vi "LVClass_WavefrontCorrector set all WFC parameter values.vi"(0 "WavefrontCorrector in":refnum<class "WavefrontCorrector.lvclass">, 5 "AllWFCParametersValues":T1[](array[typedef]), 11 "error in (no error)":errorcluster) -> (4 "WavefrontCorrector out":refnum<class "WavefrontCorrector.lvclass">, 15 "error out":errorcluster)   [LabVIEW 2020, in "WavefrontCorrector.lvclass"]
uses:
  WavefrontCorrector.lvclass
  CameraParametersSetup.ctl
  CameraParameters_Type.ctl
  LVClass_WavefrontCorrector Read AllWavefrontCorrectorParametersProperties.vi
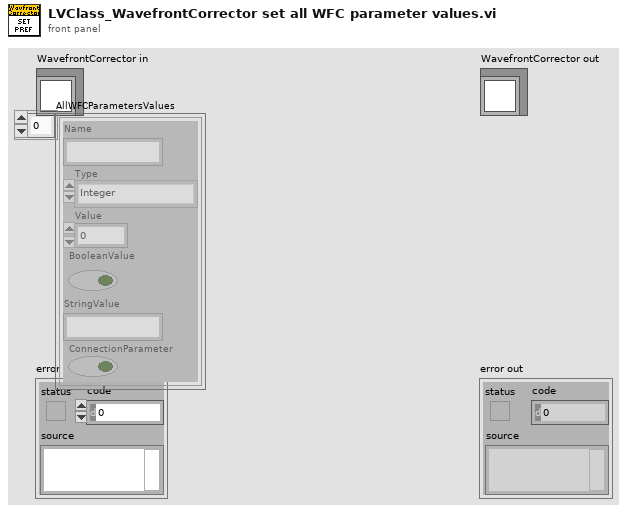
[diagram p1: front panel]
types:
  T1 = typedef "CameraParametersSetup.ctl" = cluster{"Name":string, "Type":T2, "Value":dbl, "BooleanValue":bool, "StringValue":string, "ConnectionParameter":bool}
  T2 = typedef "CameraParameters_Type.ctl" = enum16{"Integer", "Real", "String", "Boolean"}
  T3 = typedef "ParameterID.ctl" = cluster{"Name":string, "ConnectionParameter?":bool, "Type":T2, "Authorization":T4, "OnFlyAuthorization":T5, "StringValue":string, "Value":dbl, "Min":dbl, "Max":dbl, "BooleanValue":bool, "StringParameterList":string[]}
  T4 = typedef "CameraParameters_Authorization.ctl" = enum16{"Disable", "Gettable", "Settable - Gettable"}
  T5 = typedef "CameraParameters_OnFlyAuthorization.ctl" = enum16{"None", "Gettable", "Settable", "Settable - Gettable"}
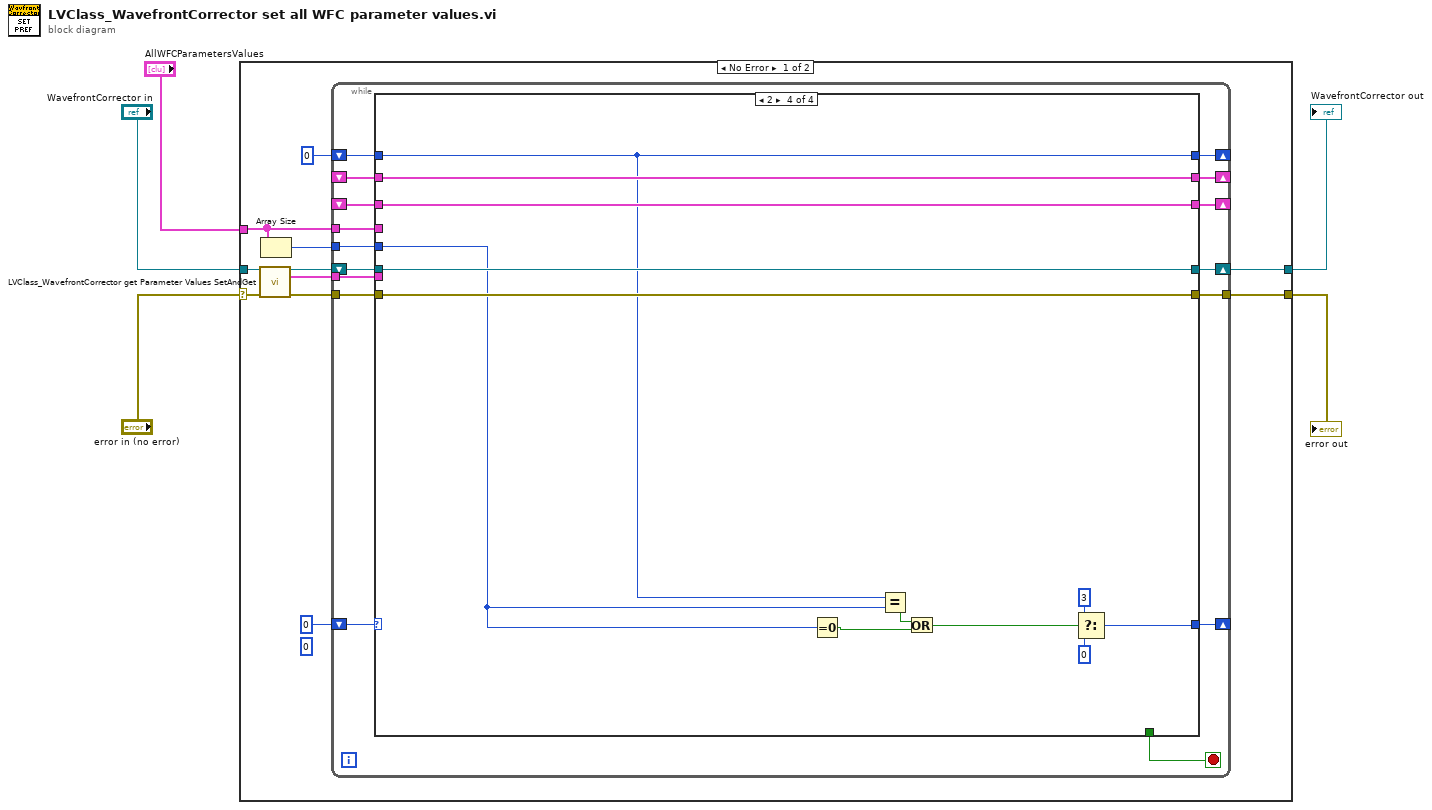
[diagram p0: block diagram]
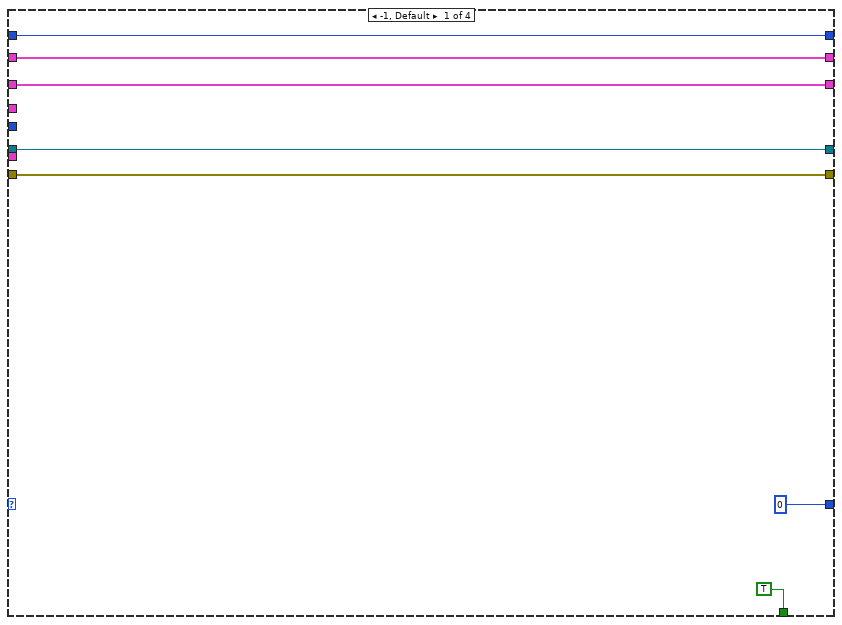
[diagram p2: hidden frame]
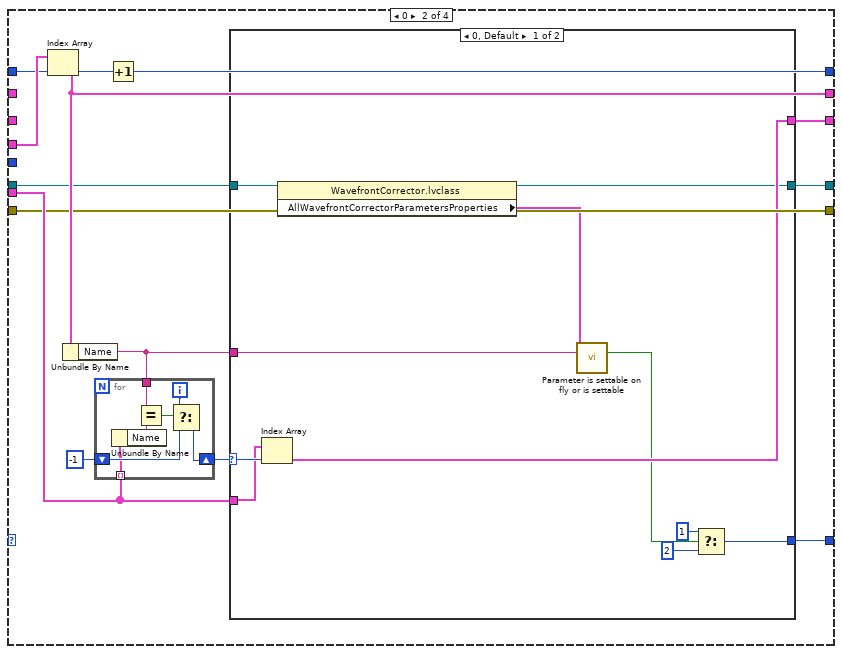
[diagram p3: hidden frame]
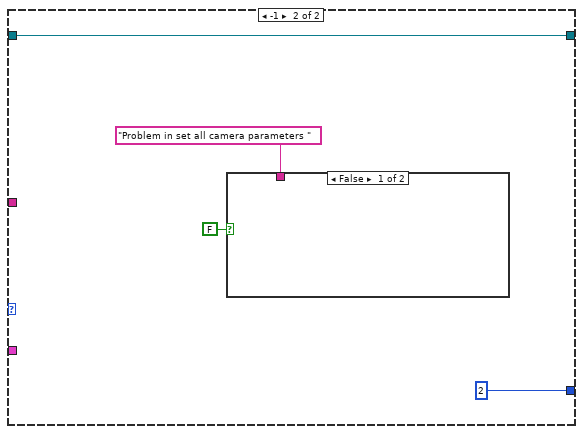
[diagram p4: hidden frame]
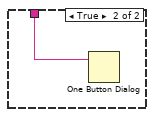
[diagram p5: hidden frame]
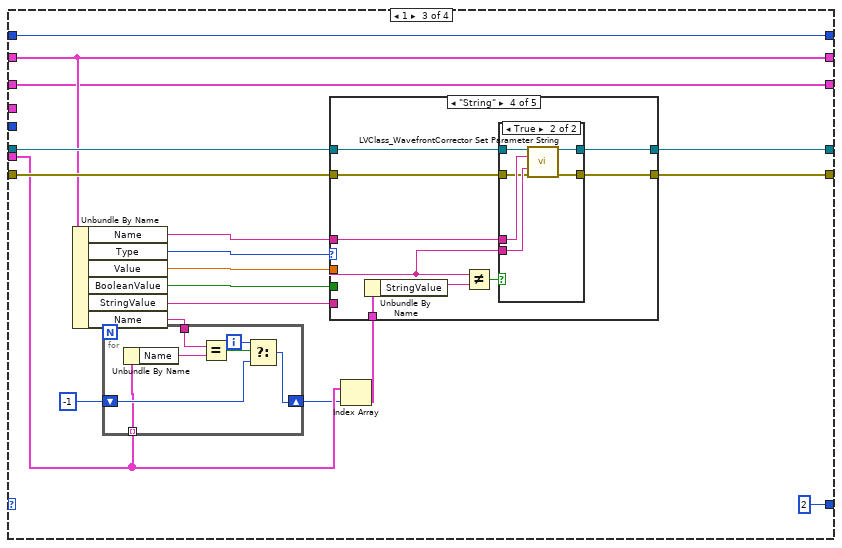
[diagram p6: hidden frame]
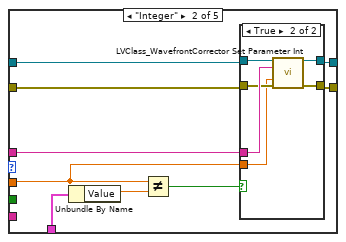
[diagram p8: hidden frame]
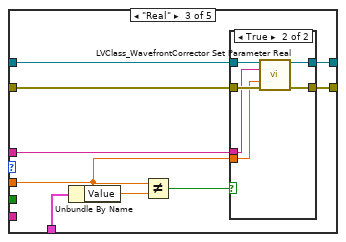
[diagram p10: hidden frame]
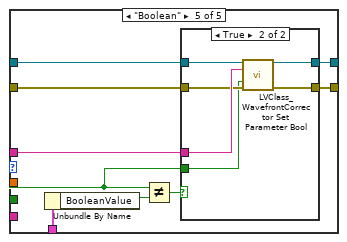
[diagram p13: hidden frame]
diagram:
  n1 = case shown="No Error" "error in (no error)" {
    selector: "error in (no error)" -> [w16 w184]
    tunnel: [w9 w184] -> w2
    tunnel: [w11 w183] -> w3
    tunnel: "WavefrontCorrector in" -> [w15 w183]
    tunnel: "AllWFCParametersValues" -> [w7 _]
    frame No Error {
      (unwired) 0
      n2 = call "LVClass_WavefrontCorrector get Parameter Values SetAndGet.vi"("WavefrontCorrector in"=w15, "error in (no error)"=w16) -> ("WavefrontCorrector out"=w12:refnum<class "WavefrontCorrector.lvclass">, "ListOfSettableAndGettableValue"=w10:T1[], "error out"=w14:errorcluster)  [unwired: 11 in]
      n3 = Array Size(array=w7) -> (size(s)=w6:i32)
      n4 = while {
        tunnel: w14 -> [w28]
        shift-right: [w31] -> _
        shift-left: 0 -> [w32]
        tunnel: w10 -> [w26]
        tunnel: [w27] -> w9
        tunnel: w7 -> [w25]
        shift-right: [w29] -> w11
        shift-left: w12 -> [w30]
        shift-right: [w20] -> _
        shift-left: 0 -> [w23]
        shift-right: [w22] -> _
        shift-left: _ -> [w21]
        tunnel: w6 -> [w19]
        shift-right: [w18] -> _
        shift-left: _ -> [w17]
        stop <- w24 stop-if-true
        n5 = case shown="2" w32 {
          tunnel: [0 w45 2 w177] -> w31
          tunnel: w30 -> [w39 w44 w92 w180]
          tunnel: [w39 w40 w91 w180] -> w29
          tunnel: w28 -> [w38 w47 w90 w179]
          tunnel: [w38 w47 w89 w179] -> w27
          tunnel: w26 -> [_ w52 w88 _]
          tunnel: w25 -> [_ w49 _ _]
          tunnel: [TRUE _ _ _] -> w24
          tunnel: w23 -> [w33 w46 w78 w178]
          tunnel: [w35 w48 w87 w182] -> w22
          tunnel: w21 -> [w35 _ w87 w182]
          tunnel: [w33 w42 w78 w178] -> w20
          tunnel: w19 -> [_ _ _ w174]
          tunnel: [w34 w41 w76 w181] -> w18
          tunnel: w17 -> [w34 _ w76 w181]
          frame -1, Default {
          }
          frame 0 {
            n6 = Index Array(array=w49, index=w46) -> (element=w48:T1)
            n7 = Unbundle By Name(w48) -> ("Name"=w43:string)
            n8 = for {
              tunnel: w43 -> [w74]
              shift-right: [w71] -> w50
              shift-left: -1 -> [w70]
              tunnel: w52 -> [w69] mode=indexing
              i -> [w72]
              n9 = Unbundle By Name(w69) -> ("Name"=w75:string)
              n10 = Equal?(x=w74, y=w75) -> (x = y?=w73:bool)
              n11 = Select(t=w72, s=w73, f=w70) -> (s? t:f=w71:i32)
            }
            n12 = Increment(x=w46) -> (x+1=w42:i32)
            n13 = case shown="0, Default" w50 {
              selector: w50 -> [w62 _]
              tunnel: w52 -> [w61 _]
              tunnel: [w63 2] -> w45
              tunnel: w44 -> [w55 w64]
              tunnel: w43 -> [w59 _]
              tunnel: [w60 _] -> w41
              tunnel: [w53 w64] -> w40
              frame 0, Default {
                n14 = Index Array(array=w61, index=w62) -> (element=w60:T1)
                n15 = property class="WavefrontCorrector.lvclass"(reference=w55) -> (reference out=w53:refnum<class "WavefrontCorrector.lvclass">, "AllWavefrontCorrectorParametersProperties"=w54:T3[])  [unwired: 1 in, 1 out]
                n16 = call "Parameter is settable on fly or is settable.vi"("AllCameraParameters"=w54, "Name"=w59) -> ("Settable?"=w56:bool)  [unwired: 11 in, 2 out]
                n17 = Select(t=1, s=w56, f=2) -> (s? t:f=w63:i32)
              }
              frame -1 {
                n18 = case shown="False" FALSE {
                  tunnel: "Problem in set all camera parameters " ("message") -> [_ w68]
                  frame False {
                  }
                  frame True {
                    n19 = One Button Dialog(message=w68) -> ()  [unwired: 1 in, 1 out]
                  }
                }
              }
            }
          }
          frame 1 {
            n20 = Unbundle By Name(w87) -> ("Name"=w81:string, "Type"=w86:T2, "Value"=w82:dbl, "BooleanValue"=w84:bool, "StringValue"=w83:string, "Name"=w80:string)
            n21 = for {
              tunnel: w80 -> [w169]
              shift-right: [w166] -> w79
              shift-left: -1 -> [w165]
              tunnel: w88 -> [w164] mode=indexing
              i -> [w167]
              n22 = Unbundle By Name(w164) -> ("Name"=w170:string)
              n23 = Equal?(x=w169, y=w170) -> (x = y?=w168:bool)
              n24 = Select(t=w167, s=w168, f=w165) -> (s? t:f=w166:i32)
            }
            n25 = Index Array(array=w88, index=w79) -> (element=w77:T1)
            n26 = case shown="\"String\"" w86 {
              tunnel: w81 -> [_ w97 w114 w136 w153]
              tunnel: w92 -> [w95 w103 w120 w137 w154]
              tunnel: [w95 w101 w118 w134 w151] -> w91
              tunnel: [w94 w100 w117 w133 w150] -> w89
              tunnel: w90 -> [w94 w102 w119 w135 w152]
              tunnel: w77 -> [_ w104 w121 w138 w155]
              tunnel: w82 -> [_ w99 w115 _ _]
              tunnel: w84 -> [_ _ _ _ w147]
              tunnel: w83 -> [_ _ _ w130 _]
              frame Default {
              }
              frame "Integer" {
                n27 = Unbundle By Name(w104) -> ("Value"=w98:dbl)
                n28 = Not Equal?(x=w99, y=w98) -> (x != y?=w96:bool)
                n29 = case shown="True" w96 {
                  tunnel: w103 -> [w106 w112]
                  tunnel: w97 -> [_ w111]
                  tunnel: w102 -> [w105 w110]
                  tunnel: [w106 w109] -> w101
                  tunnel: [w105 w108] -> w100
                  tunnel: w99 -> [_ w107]
                  frame False {
                  }
                  frame True {
                    n30 = call "LVClass_WavefrontCorrector Set Parameter Int.vi"("WavefrontCorrector in"=w112, "parameter_name"=w111, "value"=w107, "error in (no error)"=w110) -> ("WavefrontCorrector out"=w109:refnum<class "WavefrontCorrector.lvclass">, "error out"=w108:errorcluster)  [unwired: 10 in]
                  }
                }
              }
              frame "Real" {
                n31 = Unbundle By Name(w121) -> ("Value"=w116:dbl)
                n32 = Not Equal?(x=w115, y=w116) -> (x != y?=w113:bool)
                n33 = case shown="True" w113 {
                  tunnel: w120 -> [w123 w129]
                  tunnel: w114 -> [_ w125]
                  tunnel: w119 -> [w122 w126]
                  tunnel: [w123 w128] -> w118
                  tunnel: [w122 w127] -> w117
                  tunnel: w115 -> [_ w124]
                  frame False {
                  }
                  frame True {
                    n34 = call "LVClass_WavefrontCorrector Set Parameter Real.vi"("WavefrontCorrector in"=w129, "parameter_name"=w125, "value"=w124, "error in (no error)"=w126) -> ("WavefrontCorrector out"=w128:refnum<class "WavefrontCorrector.lvclass">, "error out"=w127:errorcluster)  [unwired: 10 in]
                  }
                }
              }
              frame "String" {
                n35 = Unbundle By Name(w138) -> ("StringValue"=w131:string)
                n36 = Not Equal?(x=w130, y=w131) -> (x != y?=w132:bool)
                n37 = case shown="True" w132 {
                  tunnel: w137 -> [w140 w146]
                  tunnel: w136 -> [_ w143]
                  tunnel: w135 -> [w139 w141]
                  tunnel: [w140 w145] -> w134
                  tunnel: [w139 w144] -> w133
                  tunnel: w130 -> [_ w142]
                  frame False {
                  }
                  frame True {
                    n38 = call "LVClass_WavefrontCorrector Set Parameter String.vi"("WavefrontCorrector in"=w146, "parameter_name"=w143, "value"=w142, "error in (no error)"=w141) -> ("WavefrontCorrector out"=w145:refnum<class "WavefrontCorrector.lvclass">, "error out"=w144:errorcluster)  [unwired: 10 in]
                  }
                }
              }
              frame "Boolean" {
                n39 = Unbundle By Name(w155) -> ("BooleanValue"=w148:bool)
                n40 = Not Equal?(x=w147, y=w148) -> (x != y?=w149:bool)
                n41 = case shown="True" w149 {
                  tunnel: w154 -> [w157 w163]
                  tunnel: w153 -> [_ w161]
                  tunnel: w152 -> [w156 w160]
                  tunnel: [w157 w162] -> w151
                  tunnel: [w156 w159] -> w150
                  tunnel: w147 -> [_ w158]
                  frame False {
                  }
                  frame True {
                    n42 = call "LVClass_WavefrontCorrector Set Parameter Bool.vi"("WavefrontCorrector in"=w163, "parameter_name"=w161, "value"=w158, "error in (no error)"=w160) -> ("WavefrontCorrector out"=w162:refnum<class "WavefrontCorrector.lvclass">, "error out"=w159:errorcluster)  [unwired: 10 in]
                  }
                }
              }
            }
          }
          frame 2 {
            n43 = Equal To 0?(x=w174) -> (x = 0?=w173:bool)
            n44 = Equal?(x=w178, y=w174) -> (x = y?=w172:bool)
            n45 = Or(x=w172, y=w173) -> (x .or. y?=w171:bool)
            n46 = Select(t=3, s=w171, f=0) -> (s? t:f=w177:i32)
          }
        }
      }
    }
    frame Error {
    }
  }
  "error out" <- w2
  "WavefrontCorrector out" <- w3
